vi "Write Topology to Temporary File.vi"(8 "error in (no error)":errorcluster, 11 "Topology in":T1) -> (0 "error out":errorcluster, 3 "file path":path)   [LabVIEW 2016, in "SLSC Switch.lvlib" / "SLSC Switch.lvclass"]
uses:
  SLSC Switch.lvclass
  Controls/Topology.ctl
  Controls/JSON.InitialState.ctl
  Controls/JSON.ChannelList.ctl
  Controls/JSON.ConnectionList.ctl
  <vilib>/SLSC/Flatten Names (String).vi
  <vilib>/Utility/config.llb/Write Key (String).vi
  <vilib>/Utility/config.llb/NI_LVConfig.lvlib
  <vilib>/SLSC/SLSC.lvlib
  slscsl/slscsl.lvclass
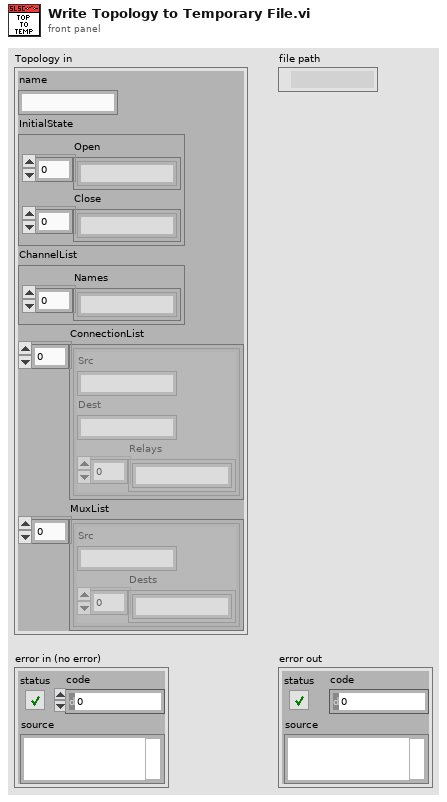
[diagram p1: front panel]
types:
  T1 = typedef "SLSC Switch.lvlib/SLSC Switch.lvclass/Topology.ctl" = cluster{"name":string, "InitialState":T2, "ChannelList":T3, "ConnectionList":T4[], "MuxList":cluster{"Src":string, "Dests":string[]}[]}
  T2 = typedef "SLSC Switch.lvlib/SLSC Switch.lvclass/JSON.InitialState.ctl" = cluster{"Open":string[], "Close":string[]}
  T3 = typedef "SLSC Switch.lvlib/SLSC Switch.lvclass/JSON.ChannelList.ctl" = cluster{"Names":string[]}
  T4 = typedef "SLSC Switch.lvlib/SLSC Switch.lvclass/JSON.ConnectionList.ctl" = cluster{"Src":string, "Dest":string, "Relays":string[]}
  T5 = typedef "NI_LVConfig.lvlib/Config Data RefNum.ctl" = refnum<k1>
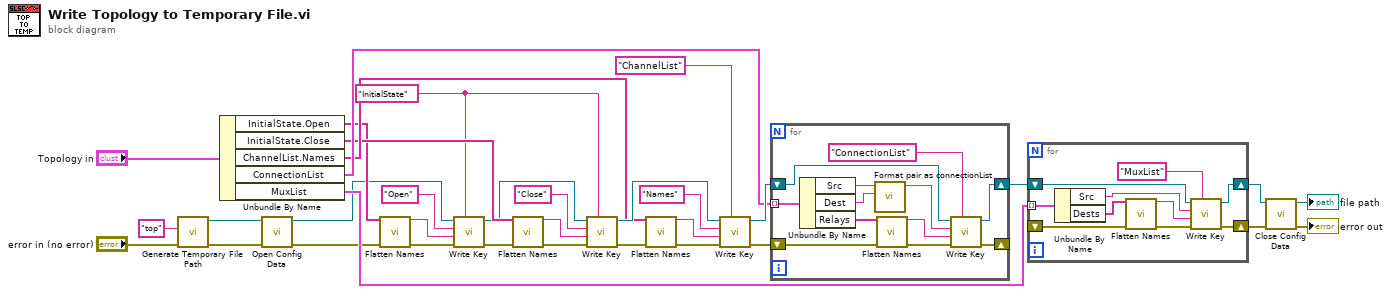
[diagram p0: block diagram]
diagram:
  w10 = "InitialState" ("section")
  n1 = call <vilib>:"Generate Temporary File Path.vi"("error in (no error)"="error in (no error)", "Temporary File Extension (tmp)"="top") -> ("error out"=w17:errorcluster, "Unique Temporary File Path"=w2:path)  [unwired: 8 in]
  n2 = Unbundle By Name("Topology in") -> ("InitialState.Open"=w5:string[], "InitialState.Close"=w12:string[], "ChannelList.Names"=w19:string[], "ConnectionList"=w25:T4[], "MuxList"=w29:cluster{"Src":string, "Dests":string[]}[])
  n3 = call <vilib>:"Open Config Data.vi"("error in (no error)"=w17, "configuration file path"=w2) -> ("error out"=w16:errorcluster, "refnum"=w4:T5)  [unwired: 7 in, 1 out]
  n4 = call-poly <vilib>:"Flatten Names.vi"("names in"=w5, "error in (no error)"=w16) -> ("names out"=w7:string, "error out"=w13:errorcluster)  [unwired: 12 in]
  n5 = call-poly <vilib>:"Write Key.vi"("section"=w10, "error in (no error)"=w13, "value"=w7, "key"="Open", "refnum"=w4) -> ("error out"=w15:errorcluster, "refnum out"=w8:T5)  [unwired: 4 in, 1 out]
  n6 = call-poly <vilib>:"Flatten Names.vi"("names in"=w12, "error in (no error)"=w15) -> ("names out"=w11:string, "error out"=w14:errorcluster)  [unwired: 12 in]
  n7 = call-poly <vilib>:"Write Key.vi"("section"=w10, "error in (no error)"=w14, "value"=w11, "key"="Close", "refnum"=w8) -> ("error out"=w18:errorcluster, "refnum out"=w20:T5)  [unwired: 4 in, 1 out]
  n8 = call-poly <vilib>:"Flatten Names.vi"("names in"=w19, "error in (no error)"=w18) -> ("names out"=w22:string, "error out"=w21:errorcluster)  [unwired: 12 in]
  n9 = call-poly <vilib>:"Write Key.vi"("section"="ChannelList", "error in (no error)"=w21, "value"=w22, "key"="Names", "refnum"=w20) -> ("error out"=w27:errorcluster, "refnum out"=w26:T5)  [unwired: 4 in, 1 out]
  n10 = for {
    tunnel: w25 -> [w44] mode=indexing
    shift-right: [w35] -> _
    shift-left: w27 -> [w37]
    shift-right: [w38] -> w28
    shift-left: w26 -> [w40]
    n11 = Unbundle By Name(w44) -> ("Src"=w45:string, "Dest"=w46:string, "Relays"=w41:string[])
    n12 = call "Format pair as connectionList.vi"("channel in"=w46, "channel 1"=w45) -> ("connectionList"=w43:string)  [unwired: 9 in]
    n13 = call-poly <vilib>:"Flatten Names.vi"("names in"=w41, "error in (no error)"=w37) -> ("names out"=w42:string, "error out"=w36:errorcluster)  [unwired: 12 in]
    n14 = call-poly <vilib>:"Write Key.vi"("section"="ConnectionList", "error in (no error)"=w36, "value"=w42, "key"=w43, "refnum"=w40) -> ("error out"=w35:errorcluster, "refnum out"=w38:T5)  [unwired: 4 in, 1 out]
  }
  n15 = for {
    tunnel: w29 -> [w55] mode=indexing
    shift-right: [w48] -> w30
    shift-left: _ -> [w50]
    shift-right: [w51] -> w31
    shift-left: w28 -> [w53]
    n16 = Unbundle By Name(w55) -> ("Src"=w56:string, "Dests"=w47:string[])
    n17 = call-poly <vilib>:"Flatten Names.vi"("names in"=w47, "error in (no error)"=w50) -> ("names out"=w54:string, "error out"=w49:errorcluster)  [unwired: 12 in]
    n18 = call-poly <vilib>:"Write Key.vi"("section"="MuxList", "error in (no error)"=w49, "value"=w54, "key"=w56, "refnum"=w53) -> ("error out"=w48:errorcluster, "refnum out"=w51:T5)  [unwired: 4 in, 1 out]
  }
  n19 = call <vilib>:"Close Config Data.vi"("error in (no error)"=w30, "refnum"=w31) -> ("error out"=→"error out":errorcluster, "file path"=→"file path":path)  [unwired: 8 in]
